vi "myTCP-client.vi"() -> ()   [LabVIEW 2024]
panel:
  out "*(type *) &x":dbl[](array[numeric])
  out "Waveform Graph":dbl[](graph)
  in  "Server Closed":string="The server VI closed the connection."
  in  "Stop":bool
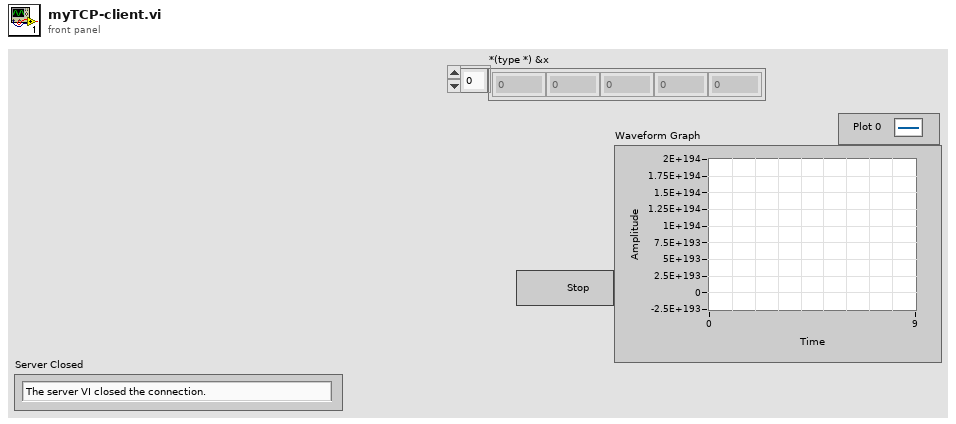
[diagram p1: front panel]
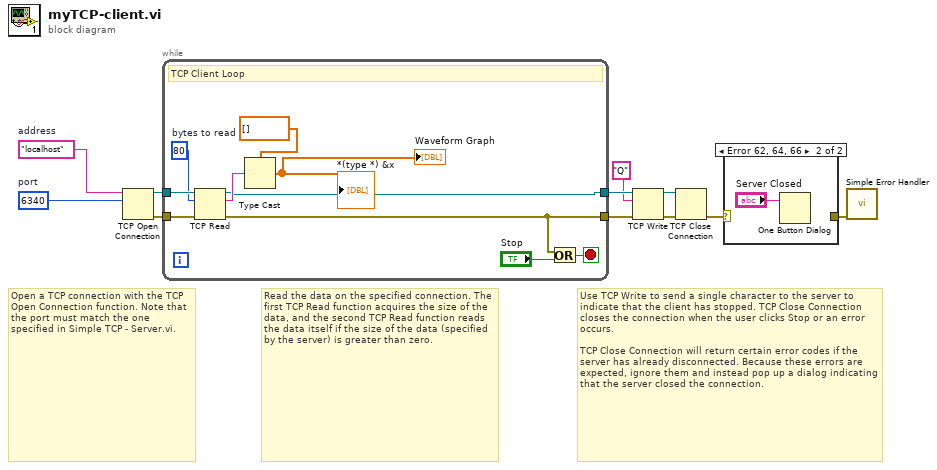
[diagram p0: block diagram]
diagram:
  w1 = u16 6340  # port
  w2 = "localhost"  # address
  # "Use TCP Write to send a single character to the server to indicate that the client has stopped. TCP Close Connection closes the connection when the user clicks Stop or an error occurs.\n\nTCP Close Connection will return certain error codes if the server has already disconnected. Because these errors are expected, ignore them and instead pop up a dialog indicating that the server closed the connection."
  # "Read the data on the specified connection. The first TCP Read function acquires the size of the data, and the second TCP Read function reads the data itself if the size of the data (specified by the server) is greater than zero."
  # "Open a TCP connection with the TCP Open Connection function. Note that the port must match the one specified in Simple TCP - Server.vi."
  n1 = TCP Open Connection(address=w2, remote port or service name=w1) -> (connection ID=w11:refnum<k5>, error out=w10:errorcluster)  [unwired: 3 in]
  n2 = while {
    tunnel: w10 -> [w19]
    tunnel: w11 -> [w20]
    tunnel: [w12] -> w8
    tunnel: [w13] -> w6
    stop <- w16 stop-if-true
    w18 = 80  # bytes to read
    # "TCP Client Loop"
    n3 = TCP Read(connection ID=w20, bytes to read=w18, error in (no error)=w19) -> (connection ID out=w12:refnum<k5>, data out=w21:string, error out=w13:errorcluster)  [unwired: 2 in]
    n4 = Type Cast(type=dbl[] [] ("chart"), x=w21) -> (*(type *) &x=→"Waveform Graph" →"*(type *) &x":dbl[])
    n5 = Or(x=w13, y="Stop") -> (x .or. y?=w16:bool)
  }
  n6 = TCP Write(connection ID=w8, data in="Q", error in (no error)=w6) -> (connection ID out=w9:refnum<k5>, error out=w7:errorcluster)  [unwired: 2 out]
  n7 = TCP Close Connection(connection ID=w9, error in (no error)=w7) -> (error out=w4:errorcluster)  [unwired: 1 in, 1 out]
  n8 = case shown="Error 62, 64, 66" w4 {
    selector: w4 -> [w22 _]
    tunnel: [w22 _] -> w3
    frame #0 {
    }
    frame #1 {
      n9 = One Button Dialog(message="Server Closed") -> ()  [unwired: 1 in, 1 out]
    }
  }
  n10 = call <vilib>:"Simple Error Handler.vi"("error in (no error)"=w3) -> ()  [unwired: 4 in, 5 out]
